vi "Test Get Debug Log Not Filtered by Inacitve Is Receive.vi"(8 "error in (no error)":errorcluster, 11 "Test Case In":refnum<class "Debugger Test.lvclass">) -> (0 "error out":errorcluster, 3 "Test Case Out":refnum<class "Debugger Test.lvclass">)   [LabVIEW 2020, in "Debugger Test.lvclass"]
uses:
  Debugger Test.lvclass
  C:/Program Files (x86)/National Instruments/LabVIEW 2020/vi.lib/Astemes/LUnit/Test Case.lvclass
  source/Debugger/Debugger.lvclass
  C:/Users/anton/Documents/GitHub/triarc-debugger/source/Process/Debug Process.lvclass
  source/Debug Data/Raw Debug Data.ctl
  source/Debug Data/Debug Data.lvclass/Debug Data.ctl
  source/Process/Debug Process.lvclass/Debug Process.ctl
  <vilib>/Astemes/LUnit/Test Case.lvclass/Test Case.ctl
  <vilib>/Astemes/LUnit/LUnit Assertion Result.lvclass/LUnit Assertion Result.ctl
  <vilib>/Astemes/LUnit/LUnit Test Case Result.lvclass/LUnit Test Case Result.ctl
  <vilib>/Astemes/LUnit/LUnit Method Result.lvclass/LUnit Method Result.ctl
  01074fa8-ee8a-411d-bc8b-fc92c4f90959.vi
  <vilib>/AdvancedString/Delimited String to 1D String Array.vi
  source/Process/Public/Lifecycle/Get Lifecycle State.vi
  <vilib>/Astemes/Triarc Framework/Broadcast Event Helpers/Execution timer.vi
  source/Process/Private/SubVIs/Wait for finish.vi
  source/Process/Protected/Messaging/Enqueue Message.vi
  source/Process/Private/SubVIs/Set Lifecycle State.vi
  <vilib>/Astemes/LUnit/Palette/Pass.vi
  <vilib>/Astemes/LUnit/Palette/Fail.vi
  <vilib>/Astemes/LUnit/Compare Variants.vi
  <vilib>/Astemes/LUnit/Describe Comparison.vi
  <vilib>/Astemes/LUnit/Set Assertion Type.vi
  <vilib>/Utility/error.llb/Clear Errors.vi
  <vilib>/Astemes/LUnit/Add test result.vi
  <vilib>/Astemes/LUnit/LUnit Write Passed.vi
  <vilib>/Astemes/LUnit/LUnit Write Message.vi
  <vilib>/Astemes/LUnit/LUnit Write Description.vi
  <vilib>/Astemes/LUnit/Variant to string.vi
  <vilib>/Astemes/LUnit/LUnit Write Assertion Type.vi
  <vilib>/Astemes/LUnit/LUnit Record Assertion Result.vi
  <vilib>/Astemes/LUnit/LUnit Aggregate Assertion Results.vi
  <vilib>/Astemes/LUnit/Assertion Result/LUnit Read Status.vi
  <vilib>/Astemes/LUnit/LUnit Read Message.vi
  <vilib>/Astemes/LUnit/LUnit Read Description.vi
  <vilib>/Astemes/LUnit/Method Result/LUnit Merge Status.vi
  <vilib>/Astemes/LUnit/LUnit Concatenate result strings.vi
  <vilib>/Utility/error.llb/Error Cluster From Error Code.vi
  <vilib>/Astemes/Triarc Framework/Broadcast Event Helpers/Dequeue Broadcast Message.vi
  <vilib>/Utility/Data Type/Get Type Information.vi
  <vilib>/Utility/LVClass/Get LV Class Name.vi
  source/Debug Data/Debug Data.lvclass
  <vilib>/Astemes/LUnit/LUnit Assertion Result.lvclass
  source/Process/Debug Process.lvclass
  <vilib>/Astemes/Triarc Framework/Broadcast Event Helpers/Broadcast Event Helpers.lvlib
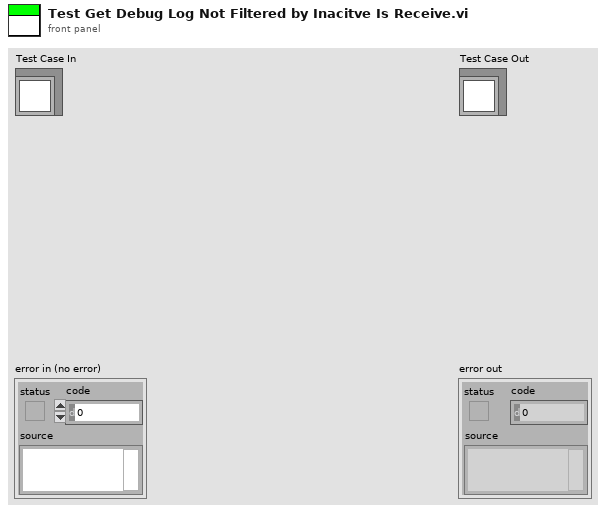
[diagram p1: front panel]
types:
  T1 = typedef "Debug Data.lvclass/Raw Debug Data.ctl" = cluster{"Action":string, "Call Chain":string, "Process":string, "Message":string, "Message Data":variant, "Time":dbl}
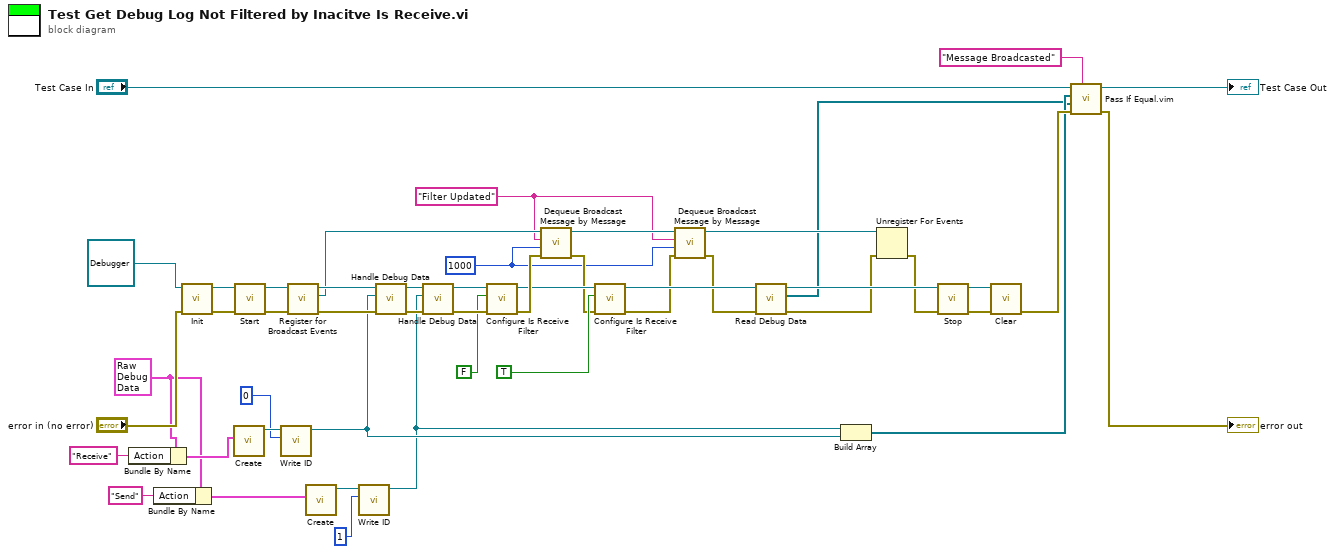
[diagram p0: block diagram]
diagram:
  w2 = "Filter Updated"
  w23 = T1 {"Action"="", "Call Chain"="", "Process"="", "Message"="", "Message Data"=variant, "Time"=0.0} ("Debug Data Cluster")
  w1 = 1000
  n1 = Bundle By Name(cluster=w23, "Action"="Receive" ("Process")) -> (w30:T1)
  n2 = Bundle By Name(cluster=w23, "Action"="Send" ("Process")) -> (w24:T1)
  n3 = call-dynamic "Init.vi"("error in (no error)"="error in (no error)", "Process In"=refnum<class "Debugger.lvclass"> refnum ("Debug Data Event In 2")) -> ("error out"=w44:errorcluster, "Process Out"=w45:refnum<class "Debugger.lvclass">)  [unwired: 8 in]
  n4 = call "Create.vi"("Debug Data Cluster"=w30) -> ("Debug Data out"=w32:refnum<class "Debug Data.lvclass">)  [unwired: 9 in, 1 out]
  n5 = call "Start.vi"("error in (no error)"=w44, "Process In"=w45) -> ("error out"=w42:errorcluster, "Process Out"=w43:refnum<class "Debugger.lvclass">)  [unwired: 7 in, 1 out]
  n6 = call "Write ID.vi"("ID"=u32 0, "Debug Data in"=w32) -> ("Debug Data out"=w13:refnum<class "Debug Data.lvclass">)  [unwired: 8 in, 1 out]
  n7 = call "Register for Broadcast Events.vi"("error in (no error)"=w42, "Process In"=w43) -> ("error out"=w41:errorcluster, "Event Registration Refnum Out"=w4:refnum<event-registration>, "Process Out"=w37:refnum<class "Debugger.lvclass">)  [unwired: 7 in]
  n8 = call "Create.vi"("Debug Data Cluster"=w24) -> ("Debug Data out"=w14:refnum<class "Debug Data.lvclass">)  [unwired: 9 in, 1 out]
  n9 = call "Write ID.vi"("ID"=u32 1, "Debug Data in"=w14) -> ("Debug Data out"=w12:refnum<class "Debug Data.lvclass">)  [unwired: 8 in, 1 out]
  n10 = call-dynamic "Handle Debug Data.vi"("error in (no error)"=w41, "Debug Data.lvclass"=w13, "Debug Data Event In"=w37) -> ("error out"=w27:errorcluster, "Debug Data Event Out"=w28:refnum<class "Debugger.lvclass">)  [unwired: 7 in]
  n11 = call-dynamic "Handle Debug Data.vi"("error in (no error)"=w27, "Debug Data.lvclass"=w12, "Debug Data Event In"=w28) -> ("error out"=w26:errorcluster, "Debug Data Event Out"=w21:refnum<class "Debugger.lvclass">)  [unwired: 7 in]
  n12 = call "Configure Is Receive Filter.vi"("error in (no error)"=w26, "Show Receive?"=FALSE ("Show Send?"), "Debugger In"=w21) -> ("error out"=w22:errorcluster, "Debugger Out"=w17:refnum<class "Debugger.lvclass">)  [unwired: 7 in]
  n13 = call <vilib>:"Dequeue Broadcast Message by Message.vi"("error in (no error)"=w22, "Timeout (-1)"=w1, "Message"=w2, "Event Registration Refnum"=w4) -> ("error out"=w5:errorcluster, "Event Registration Refnum Out"=w3:refnum<event-registration>)  [unwired: 3 in, 3 out]
  n14 = call "Configure Is Receive Filter.vi"("error in (no error)"=w5, "Show Receive?"=TRUE ("Show Send?"), "Debugger In"=w17) -> ("error out"=w8:errorcluster, "Debugger Out"=w16:refnum<class "Debugger.lvclass">)  [unwired: 7 in]
  n15 = call <vilib>:"Dequeue Broadcast Message by Message.vi"("error in (no error)"=w8, "Timeout (-1)"=w1, "Message"=w2, "Event Registration Refnum"=w3) -> ("error out"=w7:errorcluster, "Event Registration Refnum Out"=w9:refnum<event-registration>)  [unwired: 3 in, 3 out]
  n16 = call "Read Debug Data.vi"("error in (no error)"=w7, "Debugger In"=w16) -> ("error out"=w20:errorcluster, "Data Log"=w6:refnum<class "Debug Data.lvclass">[], "Debugger Out"=w40:refnum<class "Debugger.lvclass">)  [unwired: 7 in]
  n17 = Build Array(w12, w13) -> (w31:refnum<class "Debug Data.lvclass">[])
  n18 = Unregister For Events(event registration refnum=w9, error in=w20) -> (error out=w19:errorcluster)
  n19 = call "Stop.vi"("error in (no error)"=w19, "Process In"=w40) -> ("error out"=w38:errorcluster, "Process Out"=w39:refnum<class "Debugger.lvclass">)  [unwired: 7 in, 1 out]
  n20 = call-dynamic "Clear.vi"("error in (no error)"=w38, "Process In"=w39) -> ("error out"=w34:errorcluster)  [unwired: 9 in]
  n21 = call "Pass If Equal.vim"("Description"="Message Broadcasted", "error in (no error)"=w34, "Actual"=w6, "Expected"=w31, "LUnit Test Case In"="Test Case In") -> ("error out"=→"error out":errorcluster, "LUnit Test Case Out"=→"Test Case Out":refnum<class "Debugger Test.lvclass">)  [unwired: 5 in]
